vi "WriteGlobals.vi"   [LabVIEW 2019]
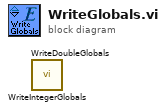
[diagram p0: block diagram]
diagram:
  n1 = call "WriteIntegerGlobals.vi"() -> ()  [unwired: 14 in, 2 out]
  n2 = call "WriteDoubleGlobals.vi"() -> ()  [unwired: 14 in, 2 out]
